vi "hexStringToByteData.vi"(9 "数据输入":string, 10 "协议":u32(ring) items=["CAN", "CANFD"]) -> (1 "CANFD_data":T1, 2 "CAN_data":T2, 3 "字节数":i32)   [LabVIEW 2018]
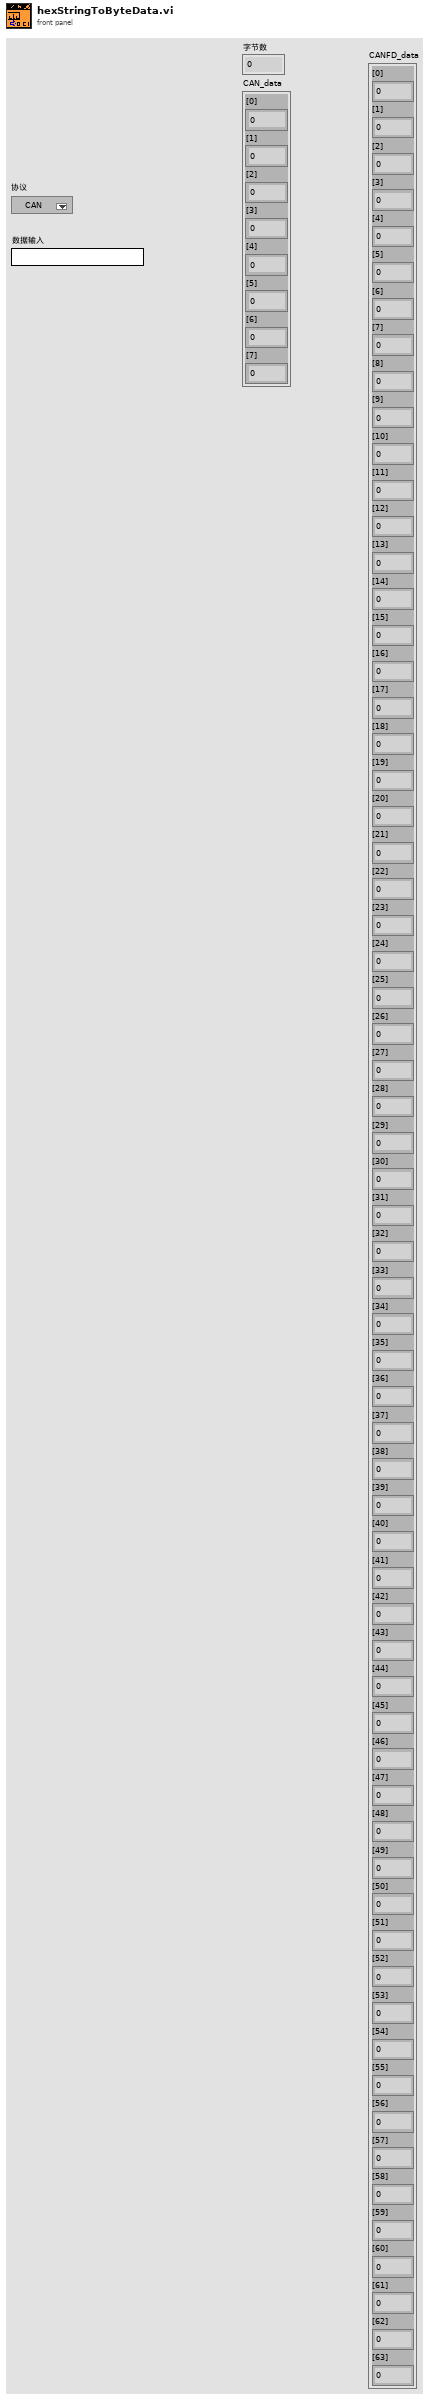
[diagram p1: front panel]
types:
  T1 = cluster{"[0]":u32, "[1]":u32, "[2]":u32, "[3]":u32, "[4]":u32, "[5]":u32, "[6]":u32, "[7]":u32, "[8]":u32, "[9]":u32, "[10]":u32, "[11]":u32, "[12]":u32, "[13]":u32, "[14]":u32, "[15]":u32, "[16]":u32, "[17]":u32, "[18]":u32, "[19]":u32, "[20]":u32, "[21]":u32, "[22]":u32, "[23]":u32, "[24]":u32, "[25]":u32, "[26]":u32, "[27]":u32, "[28]":u32, "[29]":u32, "[30]":u32, "[31]":u32, "[32]":u32, "[33]":u32, "[34]":u32, "[35]":u32, "[36]":u32, "[37]":u32, "[38]":u32, "[39]":u32, "[40]":u32, "[41]":u32, "[42]":u32, "[43]":u32, "[44]":u32, "[45]":u32, "[46]":u32, "[47]":u32, "[48]":u32, "[49]":u32, "[50]":u32, "[51]":u32, "[52]":u32, "[53]":u32, "[54]":u32, "[55]":u32, "[56]":u32, "[57]":u32, "[58]":u32, "[59]":u32, "[60]":u32, "[61]":u32, "[62]":u32, "[63]":u32}
  T2 = cluster{"[0]":u32, "[1]":u32, "[2]":u32, "[3]":u32, "[4]":u32, "[5]":u32, "[6]":u32, "[7]":u32}
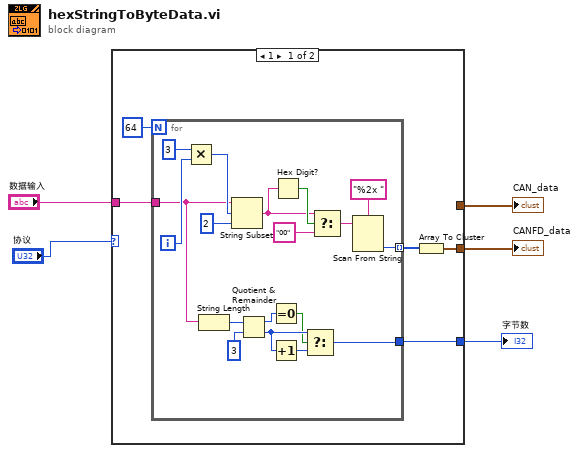
[diagram p0: block diagram]
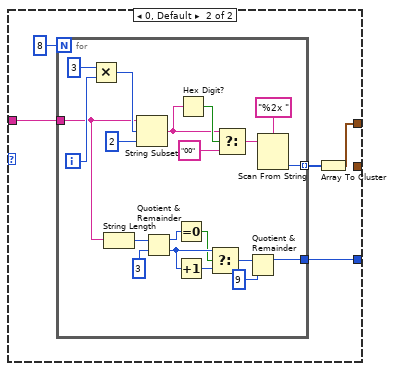
[diagram p2: hidden frame]
diagram:
  n1 = case shown="1" "协议" {
    tunnel: "数据输入" -> [w9 w33]
    tunnel: [w8 w31] -> w4
    tunnel: [_ w29] -> w2
    tunnel: [w6 _] -> w1
    frame 1 {
      n2 = for {
        N: 64 -> [_]
        tunnel: w9 -> [w13]
        tunnel: [w24] -> w7 mode=indexing
        tunnel: [w11] -> w8
        i -> [w19]
        n3 = Multiply(x=3, y=w19) -> (x*y=w27:i32)
        n4 = String Length(string=w13) -> (length=w18:i32)
        n5 = String Subset(string=w13, offset (0)=w27, length (rest)=2 ("length (rest)")) -> (substring=w21:string)
        n6 = Quotient & Remainder(x=w18, y=3) -> (x-y*floor(x/y)=w16:i32, floor(x/y)=w14:i32)
        n7 = Equal To 0?(x=w16) -> (x = 0?=w12:bool)
        n8 = Increment(x=w14) -> (x+1=w15:i32)
        n9 = Hex Digit?(1:w21) -> (0:w22:bool)
        n10 = Select(t=w14, s=w12, f=w15) -> (s? t:f=w11:i32)
        n11 = Select(t=w21, s=w22, f="00" ("t")) -> (s? t:f=w23:string)
        n12 = Scan From String(format string="%2x ", input string=w23) -> (output 1=w24:u32)  [unwired: 2 in, 4 out]
      }
      n13 = Array To Cluster(array=w7) -> (cluster=w6:T1)
    }
    frame 0, Default {
      n14 = for {
        N: 8 -> [_]
        tunnel: w33 -> [w36]
        tunnel: [w49] -> w30 mode=indexing
        tunnel: [w35] -> w31
        i -> [w44]
        n15 = Multiply(x=3, y=w44) -> (x*y=w52:i32)
        n16 = String Length(string=w36) -> (length=w43:i32)
        n17 = String Subset(string=w36, offset (0)=w52, length (rest)=2 ("length (rest)")) -> (substring=w46:string)
        n18 = Quotient & Remainder(x=w43, y=3) -> (x-y*floor(x/y)=w41:i32, floor(x/y)=w39:i32)
        n19 = Equal To 0?(x=w41) -> (x = 0?=w34:bool)
        n20 = Increment(x=w39) -> (x+1=w40:i32)
        n21 = Hex Digit?(1:w46) -> (0:w47:bool)
        n22 = Select(t=w39, s=w34, f=w40) -> (s? t:f=w38:i32)
        n23 = Select(t=w46, s=w47, f="00" ("t")) -> (s? t:f=w48:string)
        n24 = Quotient & Remainder(x=w38, y=9) -> (x-y*floor(x/y)=w35:i32)  [unwired: 1 out]
        n25 = Scan From String(format string="%2x ", input string=w48) -> (output 1=w49:u32)  [unwired: 2 in, 4 out]
      }
      n26 = Array To Cluster(array=w30) -> (cluster=w29:T2)
    }
  }
  "字节数" <- w4
  "CAN_data" <- w2
  "CANFD_data" <- w1
